vi "Delete-Window.vi"(8 "error in (no error)":errorcluster, 11 "GLF Window in":refnum<class "Window.lvclass">) -> (0 "error out":errorcluster, 3 "GLF Window out":refnum<class "Window.lvclass">)   [LabVIEW 2020, in "GLF.lvlib" / "Window.lvclass"]
uses:
  Window.lvclass
  Window.lvclass/Window.ctl
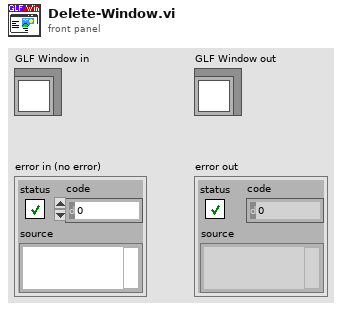
[diagram p1: front panel]
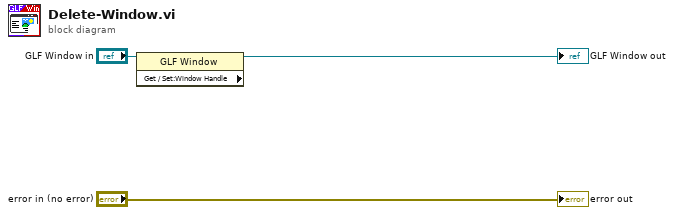
[diagram p0: block diagram]
diagram:
  n1 = property class="GLF Window" props=["Get / Set:Window Handle"](reference="GLF Window in") -> (reference out=→"GLF Window out":refnum<class "Window.lvclass">)  [unwired: 1 in, 2 out]
  "error out" <- "error in (no error)"
